vi "Build-Build Items.vi"(0 "project in":refnum<vi>, 5 "specs in":refnum<vi>[](array[refnum]), 9 "slide in":refnum<vi>, 11 "error in (no error)":errorcluster) -> (4 "project out":refnum<vi>, 10 "slide out":refnum<vi>, 15 "error out":errorcluster)   [LabVIEW 2020]
uses:
  <vilib>/AppBuilder/AB_API_Simple/Build (path).vi
  <vilib>/AppBuilder/AB_API_Simple/NI_App_Builder_API.lvlib
panel:
  in  "stop":bool
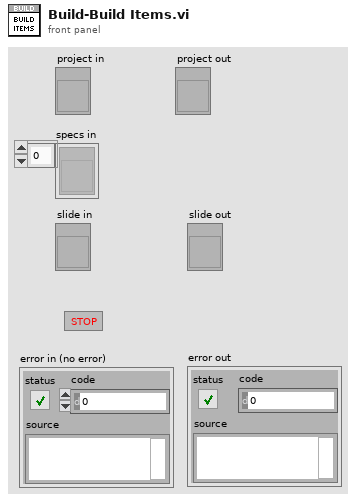
[diagram p1: front panel]
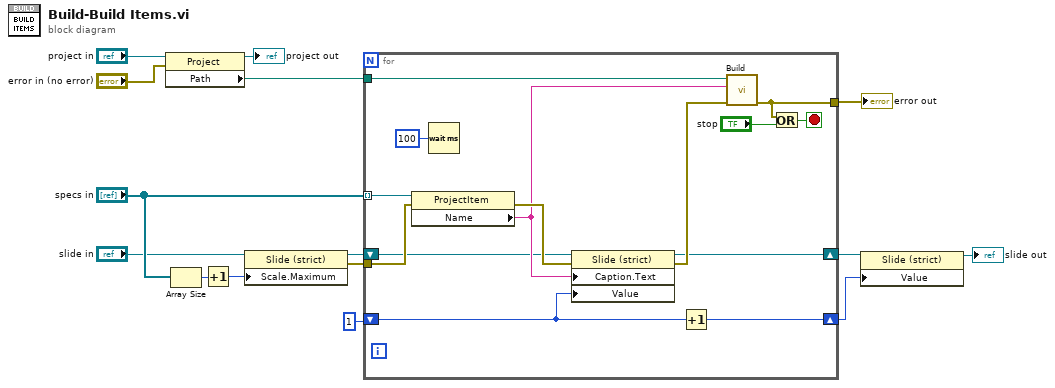
[diagram p0: block diagram]
diagram:
  n1 = property class="Project"(reference="project in", error in="error in (no error)") -> (reference out=→"project out":refnum<vi>, "Path"=w7:path)  [unwired: 1 out]
  n2 = Array Size(array="specs in") -> (size(s)=w13:i32)
  n3 = Increment(x=w13) -> (x+1=w15:i32)
  n4 = property on="Property Node" class="Slide (strict)"(reference="slide in", "Scale.Maximum"=w15) -> (reference out=w5:refnum<vi>, error out=w8:errorcluster)  [unwired: 1 in]
  n5 = for {
    tunnel: w7 -> [w29]
    tunnel: "specs in" -> [w28] mode=indexing
    tunnel: [w20] -> w10
    tunnel: w8 -> [w27]
    shift-right: [w25] -> w3
    shift-left: 1 -> [w26]
    shift-right: [w16] -> w4
    shift-left: w5 -> [w17]
    stop <- w19 stop-if-true
    n6 = property class="ProjectItem"(reference=w28, error in=w27) -> (error out=w23:errorcluster, "Name"=w22:string)  [unwired: 1 out]
    n7 = Wait (ms)(milliseconds to wait=u32 100) -> ()  [unwired: 1 out]
    n8 = property on="Property Node" class="Slide (strict)"(reference=w17, error in=w23, "Caption.Text"=w22, "Value"=w26) -> (reference out=w16:refnum<vi>, error out=w21:errorcluster)
    n9 = Increment(x=w26) -> (x+1=w25:i32)
    n10 = call-poly <vilib>:"Build.vi"("error in (no error)"=w21, "Name of build specification (if empty: build all)"=w22, "Path to project"=w29) -> ("error out"=w20:errorcluster)  [unwired: 7 in, 1 out]
    n11 = Or(x=w20, y="stop") -> (x .or. y?=w19:bool)
  }
  "error out" <- w10
  n12 = property on="Property Node" class="Slide (strict)"(reference=w4, "Value"=w3) -> (reference out=→"slide out":refnum<vi>)  [unwired: 1 in, 1 out]
